vi "Get IO Names.vi"(8 "error in (no error)":errorcluster, 11 "Module in":refnum<class "Module.lvclass">) -> (0 "error out":errorcluster, 2 "IO Names":string[](array[string]), 3 "Module out":refnum<class "Module.lvclass">)   [LabVIEW 2015, in "Module.lvclass"]
uses:
  Module.lvclass
  Module.lvclass/Module.ctl
  Signal/Signal/Read IO Name.vi
  Signal/Signal/Signal.lvclass
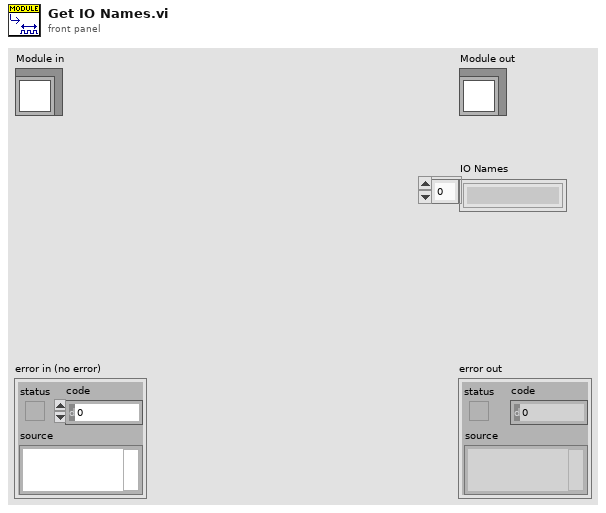
[diagram p1: front panel]
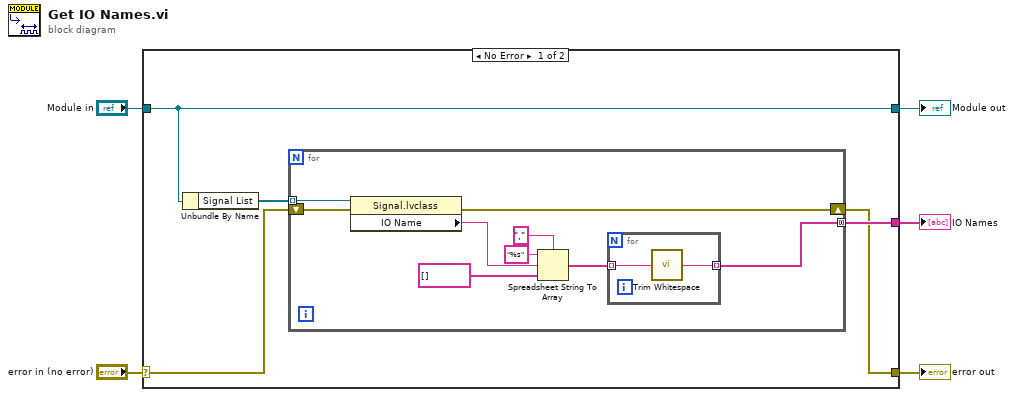
[diagram p0: block diagram]
diagram:
  n1 = case shown="No Error" "error in (no error)" {
    selector: "error in (no error)" -> [w7 w23]
    tunnel: [w6 w23] -> w4
    tunnel: [w10 w22] -> w2
    tunnel: "Module in" -> [w10 w22]
    tunnel: [w8 _] -> w1
    frame No Error {
      n2 = Unbundle By Name(w10) -> ("Signal List"=w9:refnum<class "Signal.lvclass">[])
      n3 = for {
        tunnel: w9 -> [w19] mode=indexing
        tunnel: [w11] -> w8 mode=concatenating
        shift-right: [w17] -> w6
        shift-left: w7 -> [w18]
        n4 = property class="Signal.lvclass"(reference=w19, error in=w18) -> (error out=w17:errorcluster, "IO Name"=w13:string)  [unwired: 1 out]
        n5 = Spreadsheet String To Array(delimiter (Tab)=",", format string="%s", spreadsheet string=w13, array type (2D Dbl)=string[] []) -> (array=w12:string[])
        n6 = for {
          tunnel: w12 -> [w21] mode=indexing
          tunnel: [w20] -> w11 mode=indexing
          n7 = call <vilib>:"Trim Whitespace.vi"("string"=w21) -> ("trimmed string"=w20:string)  [unwired: 1 in]
        }
      }
    }
    frame Error {
    }
  }
  "error out" <- w4
  "Module out" <- w2
  "IO Names" <- w1
